vi "SSC Digital Configure Voltage Levels.vi"(0 "Digital SSC in":T1[](array[typedef]), 1 "vol (V)":dbl format="%#_6p", 2 "voh (V)":dbl format="%#_6p", 5 "vih (V)":dbl format="%#_6p", 7 "vil (V)":dbl format="%#_6p", 9 "vterm (V)":dbl format="%#_6p", 11 "error in":errorcluster) -> (4 "Digital SSC out":T1[](array[typedef]), 15 "error out":errorcluster)   [LabVIEW 2019]
doc: "Configures voltage levels for the specified pin(s) and pin group(s)."
uses:
  SSC Digital.ctl
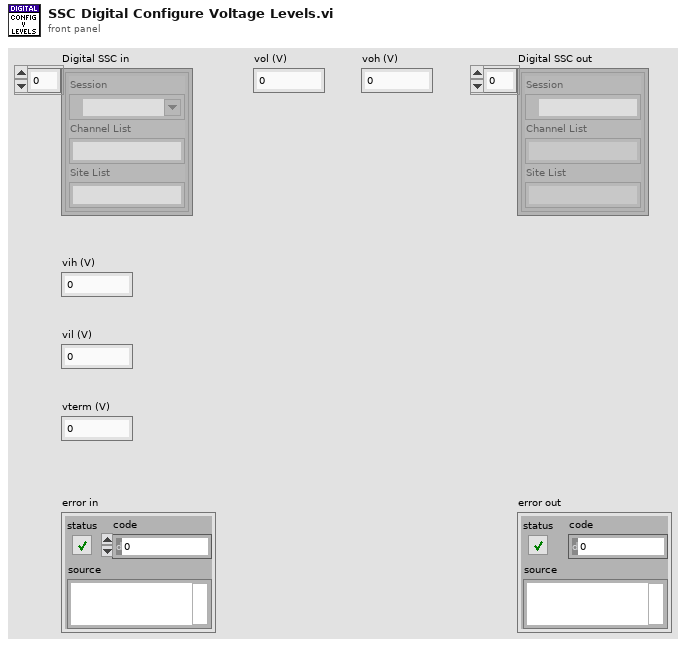
[diagram p1: front panel]
types:
  T1 = typedef "SSC Digital.ctl" = cluster{"Session":refnum<k15>, "Channel List":string, "Site List":string}
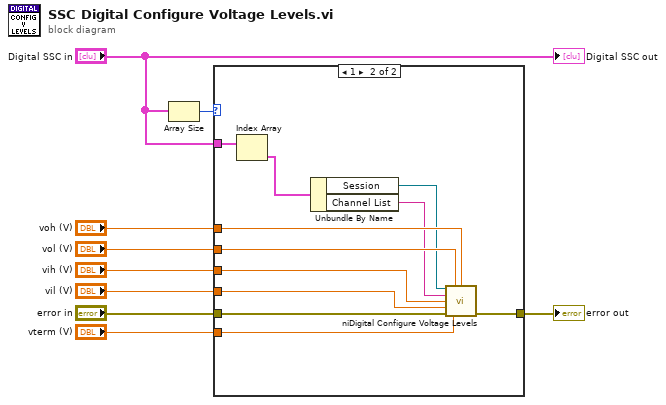
[diagram p0: block diagram]
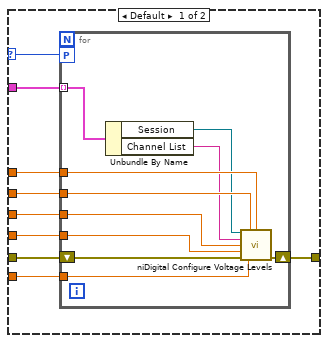
[diagram p2: hidden frame]
diagram:
  n1 = Array Size(array="Digital SSC in") -> (size(s)=w2:i32)
  n2 = case shown="1" w2 {
    selector: w2 -> [w11 _]
    tunnel: "vterm (V)" -> [w18 w39]
    tunnel: "vil (V)" -> [w17 w38]
    tunnel: "vih (V)" -> [w16 w37]
    tunnel: "vol (V)" -> [w15 w36]
    tunnel: "voh (V)" -> [w14 w35]
    tunnel: "error in" -> [w13 w34]
    tunnel: [w12 w33] -> w3
    tunnel: "Digital SSC in" -> [w10 w32]
    frame Default {
      n3 = for {
        workers-P: w11 -> [_]
        tunnel: w16 -> [w26]
        tunnel: w17 -> [w25]
        tunnel: w18 -> [w24]
        tunnel: w15 -> [w23]
        tunnel: w14 -> [w22]
        tunnel: w10 -> [w21] mode=indexing
        shift-right: [w27] -> w12
        shift-left: w13 -> [w28]
        n4 = Unbundle By Name(w21) -> ("Session"=w20:refnum<k15>, "Channel List"=w19:string)
        n5 = call <instrlib>:"niDigital Configure Voltage Levels.vi"("instrument handle"=w20, "vol (V)"=w23, "voh (V)"=w22, "channel list"=w19, "vih (V)"=w26, "vil (V)"=w25, "error in"=w28, "vterm (V)"=w24) -> ("error out"=w27:errorcluster)  [unwired: 6 in, 1 out]
      }
    }
    frame 1 {
      n6 = Index Array(array=w32) -> (element=w29:T1)  [unwired: 1 in]
      n7 = Unbundle By Name(w29) -> ("Session"=w31:refnum<k15>, "Channel List"=w30:string)
      n8 = call <instrlib>:"niDigital Configure Voltage Levels.vi"("instrument handle"=w31, "vol (V)"=w36, "voh (V)"=w35, "channel list"=w30, "vih (V)"=w37, "vil (V)"=w38, "error in"=w34, "vterm (V)"=w39) -> ("error out"=w33:errorcluster)  [unwired: 6 in, 1 out]
    }
  }
  "error out" <- w3
  "Digital SSC out" <- "Digital SSC in"
